vi "Drive Motor Control Test.vi"() -> ()   [LabVIEW 2009]
uses:
  Motor Output Global.vi
  Motor Encoder Global.vi
  Inner Control/Drive Control Global DO NOT MODIFY!.vi
panel:
  in  "Manual Override?":bool
  in  "stop":bool
  in  "Drive Speed Control Feedback Gain":fxp<+/-,20,5>
  in  "Drive Speed Set Point (ft/sec)":fxp<+/-,14,4>
  in  "Drive Enable":bool
  out "Drive Encoder ft/sec":fxp<+/-,14,4>
  out "Drive Encoder tick/count":i32
  out "Drive Encoder":i32
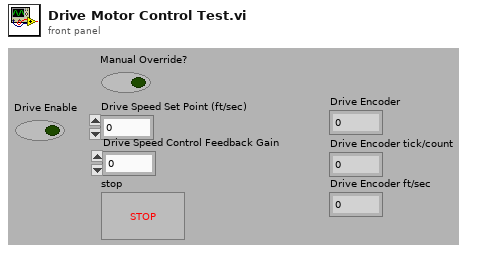
[diagram p1: front panel]
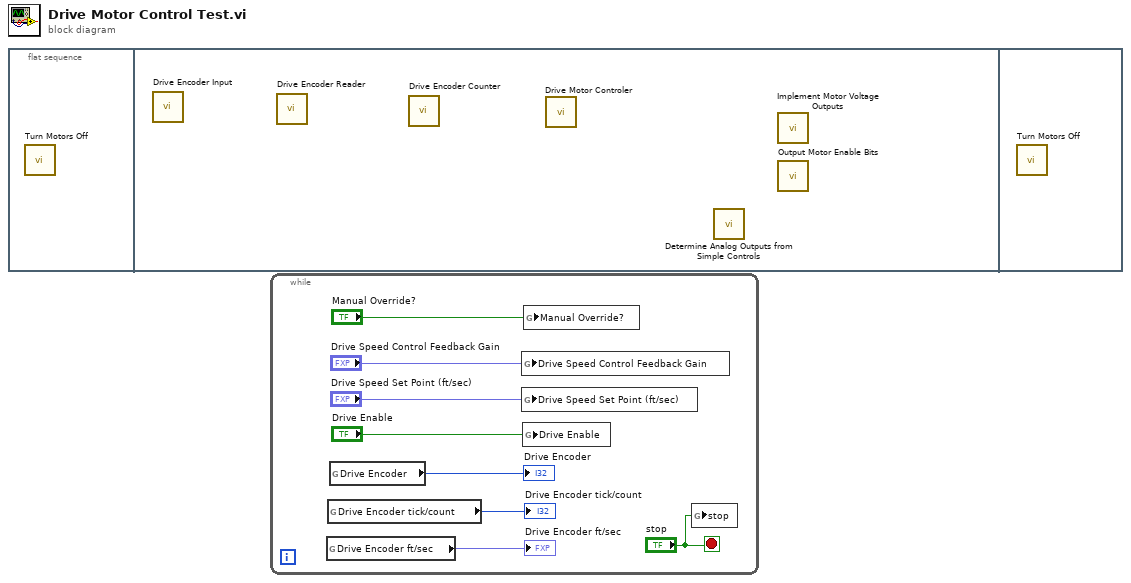
[diagram p0: block diagram]
diagram:
  n1 = flat-sequence {
    frame #0 {
      n2 = call "Turn Motors Off.vi"() -> ()  [unwired: 1 in]
    }
    frame #1 {
      n3 = call "Drive Encoder Input.vi"() -> ()  [unwired: 1 in]
      n4 = call "Drive Encoder Reader.vi"() -> ()  [unwired: 1 in]
      n5 = call "Drive Encoder Counter.vi"() -> ()  [unwired: 1 in]
      n6 = call "Drive Motor Controler.vi"() -> ()  [unwired: 1 in]
      n7 = call "Determine Analog Outputs from Simple Controls.vi"() -> ()  [unwired: 1 in]
      n8 = call "Implement Motor Voltage Outputs.vi"() -> ()  [unwired: 1 in]
      n9 = call "Output Motor Enable Bits.vi"() -> ()  [unwired: 1 in]
    }
    frame #2 {
      n10 = call "Turn Motors Off.vi"() -> ()  [unwired: 1 in]
    }
  }
  n11 = while {
    stop <- "stop" stop-if-true
    n12 = global read "Drive Control Global DO NOT MODIFY!.vi" "Drive Encoder ft/sec"() -> (→"Drive Encoder ft/sec":fxp<+/-,18,8>)
    n13 = global read "Drive Control Global DO NOT MODIFY!.vi" "Drive Encoder tick/count"() -> (→"Drive Encoder tick/count":u32)
    n14 = global read "Motor Encoder Global.vi" "Drive Encoder"() -> (→"Drive Encoder":i32)
    n15 = global write "Motor Encoder Global.vi" "Drive Speed Control Feedback Gain"("Drive Speed Control Feedback Gain") -> ()
    n16 = global write "Motor Encoder Global.vi" "Drive Speed Set Point (ft/sec)"("Drive Speed Set Point (ft/sec)") -> ()
    n17 = global write "Motor Output Global.vi" "Drive Enable"("Drive Enable") -> ()
    n18 = global write "Motor Output Global.vi" "Manual Override?"("Manual Override?") -> ()
    n19 = global write "Motor Encoder Global.vi" "stop"("stop") -> ()
  }
